vi "Create.vi"(6 "Server Certificate File (.crt)":path, 8 "error in (no error)":errorcluster, 9 "VI Reference":refnum<vi>, 10 "Manager Address":string, 11 "CIF_UI in":refnum<class "CIF_UI.lvclass">) -> (0 "error out":errorcluster, 3 "CIF_UI out":refnum<class "CIF_UI.lvclass">)   [LabVIEW 2021, in "CIF_UI.lvclass"]
uses:
  CIF_UI.lvclass
  CIF_UI.lvclass/CIF_UI.ctl
  CIFPluginManager/CIFPluginManager/gRPC/CIF_Manager_Client_Wrapper/CIFManagerClientWrapper.lvlib
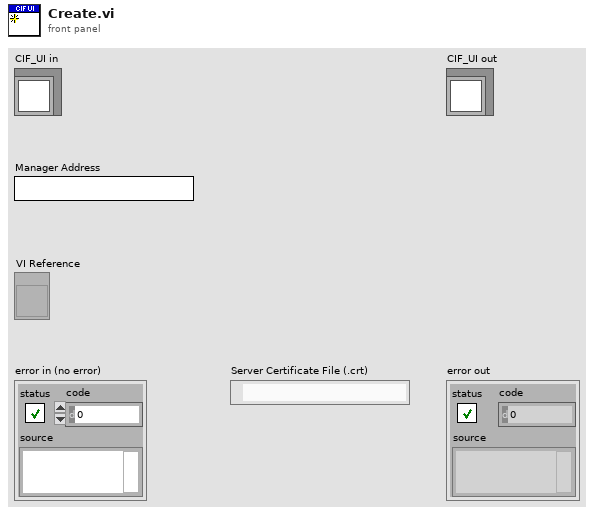
[diagram p1: front panel]
types:
  T1 = typedef "grpc-lvsupport-release.lvlib/grpcId.ctl" = u64
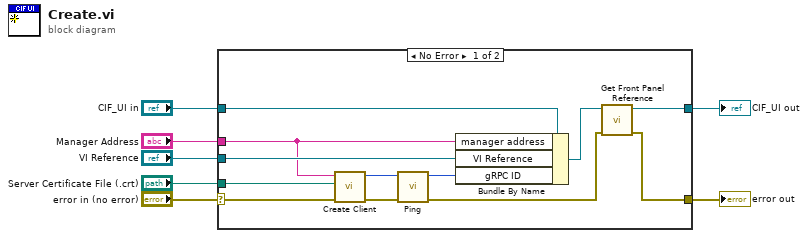
[diagram p0: block diagram]
diagram:
  n1 = case shown="No Error" "error in (no error)" {
    selector: "error in (no error)" -> [w15 w21]
    tunnel: [w14 w21] -> w6
    tunnel: [w13 w20] -> w4
    tunnel: "CIF_UI in" -> [w18 w20]
    tunnel: "Manager Address" -> [w17 _]
    tunnel: "VI Reference" -> [w19 _]
    tunnel: "Server Certificate File (.crt)" -> [w16 _]
    frame No Error {
      n2 = call "Create Client.vi"("error in"=w15, "Server Certificate File (.crt)"=w16, "address"=w17) -> ("error out"=w12:errorcluster, "gRPC ID Out"=w8:T1)  [unwired: 7 in]
      n3 = call "Ping.vi"("error in"=w12, "gRPC ID in"=w8) -> ("error out"=w11:errorcluster, "gRPC ID out"=w9:T1)  [unwired: 8 in]
      n4 = Bundle By Name(cluster=w18, "manager address"=w17, "VI Reference"=w19, "gRPC ID"=w9) -> (w10:refnum<class "CIF_UI.lvclass">)
      n5 = call "Get Front Panel Reference.vi"("error in (no error)"=w11, "CIF_UI in"=w10) -> ("error out"=w14:errorcluster, "CIF_UI out"=w13:refnum<class "CIF_UI.lvclass">)  [unwired: 8 in]
    }
    frame Error {
    }
  }
  "error out" <- w6
  "CIF_UI out" <- w4
